vi "resultsColumnsLDA.vi"(10 "chValuesIn":string[](array[string]), 11 "chNamesIn":string[](array[string])) -> (2 "chValuesOut":string[](array[string]), 3 "chNamesOut":string[](array[string]))   [LabVIEW 2020]
uses:
  Globals/Meas_global.vi
  Globals/Trav_pos_global.vi
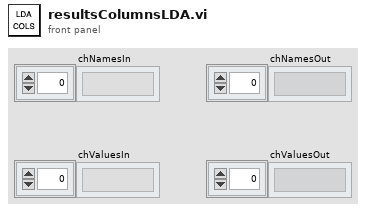
[diagram p1: front panel]
types:
  T1 = typedef "Post_Process.ctl" = enum16{"Take New Data", "Post Process Raw Data File"}
  T2 = typedef "Trigger_Mode.ctl" = enum16{"Free Running", "Start on Trigger", "Trigger Every Block", "Trigger Every Sample"}
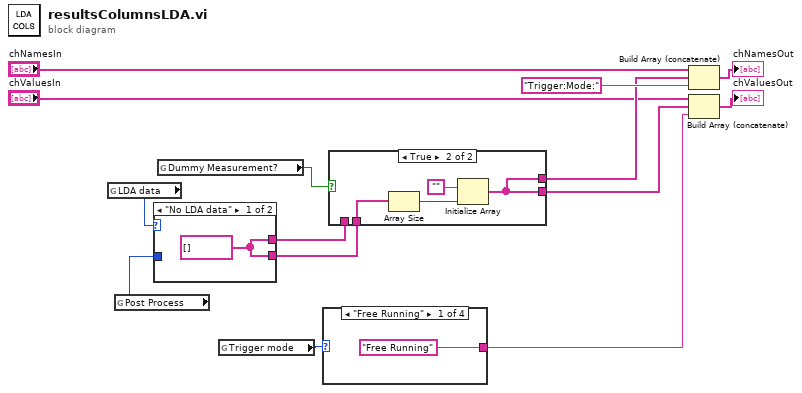
[diagram p0: block diagram]
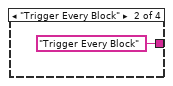
[diagram p2: hidden frame]
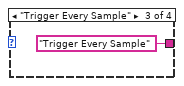
[diagram p3: hidden frame]
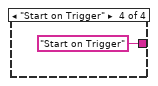
[diagram p4: hidden frame]
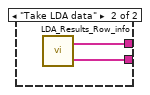
[diagram p6: hidden frame]
diagram:
  n1 = global read "Meas_global.vi" "LDA data"() -> (w13:enum16{"No LDA data", "Take LDA data"})
  n2 = global read "Meas_global.vi" "Post Process"() -> (w14:T1)
  n3 = case shown="\"No LDA data\"" w13 {
    tunnel: w14 -> [_ _]
    tunnel: [w15 w16] -> w4
    tunnel: [w15 w17] -> w5
    frame "No LDA data" {
      w15 = string[] []
    }
    frame "Take LDA data" {
      n4 = call "LDA_Results_Row_info.vi"() -> ("Row Values"=w16:string[], "Row Headers"=w17:string[])  [unwired: 2 in]
    }
  }
  n5 = global read "Trav_pos_global.vi" "Dummy Measurement?"() -> (w12:bool)
  n6 = global read "Meas_global.vi" "Trigger mode"() -> (w9:T2)
  n7 = case shown="\"Free Running\"" w9 {
    tunnel: ["Free Running" "Trigger Every Block" "Trigger Every Sample" "Start on Trigger"] -> w11
    frame "Free Running" {
    }
    frame "Trigger Every Block" {
    }
    frame "Trigger Every Sample" {
    }
    frame "Start on Trigger" {
    }
  }
  n8 = case shown="True" w12 {
    tunnel: [w23 w24] -> w3
    tunnel: w4 -> [w23 w27]
    tunnel: [w22 w24] -> w8
    tunnel: w5 -> [w22 _]
    frame False {
    }
    frame True {
      n9 = Array Size(array=w27) -> (size(s)=w26:i32)
      n10 = Initialize Array("", w26) -> (w24:string[])
    }
  }
  n11 = Build Array (concatenate)("chNamesIn", w8, "Trigger:Mode:") -> (→"chNamesOut":string[])
  n12 = Build Array (concatenate)("chValuesIn", w3, w11) -> (→"chValuesOut":string[])
